vi "PUT_gear_change.vi"(8 "API Key":string="0", 9 "Cluster":cluster{"gear":string}) -> (0 "headers":string="0\r\nContent-Length: 58\r\nConnection: close\r\n\r\n", 1 "JSON string":string="0", 2 "gear":cluster{"gear":string})   [LabVIEW 2024]
uses:
  <vilib>/httpClient/PUTBuffer.vi
  <vilib>/httpClient/LabVIEWHTTPClient.lvlib
panel:
  out "error out json":errorcluster
  out "body":string="0"
  out "error out put":errorcluster
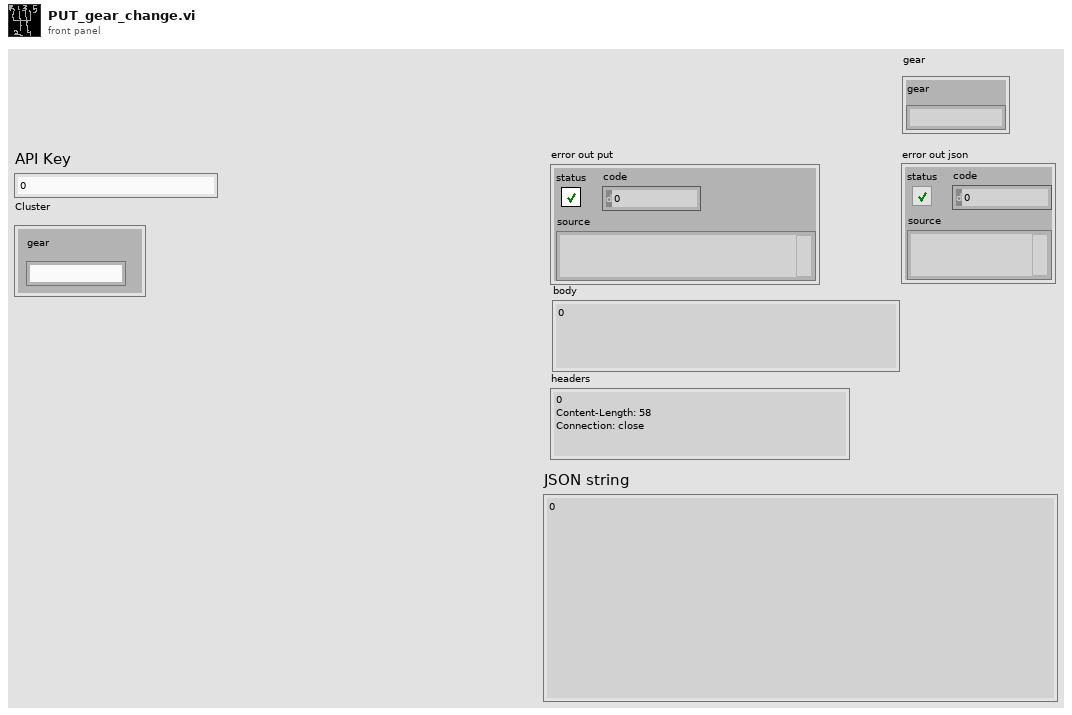
[diagram p1: front panel]
types:
  T1 = typedef "LabVIEWHTTPClient.lvlib/ClientHandle.ctl" = refnum<k1>
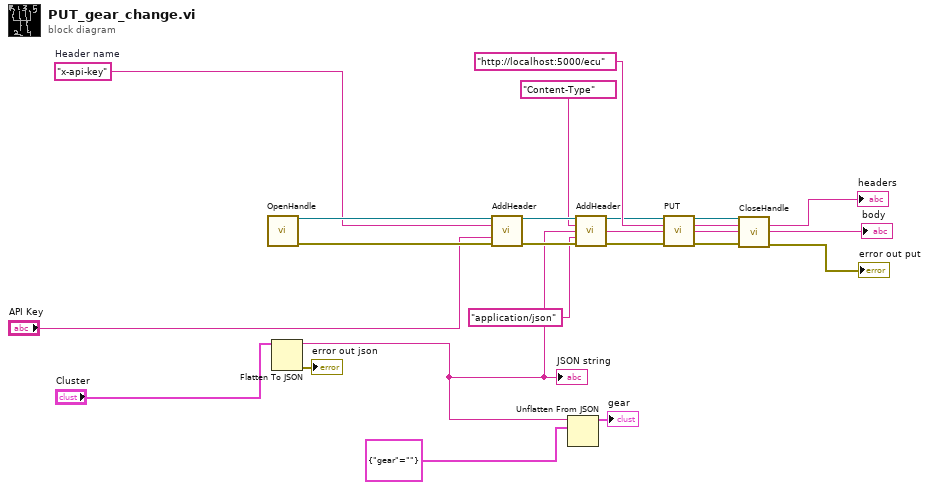
[diagram p0: block diagram]
diagram:
  w14 = "x-api-key"  # Header name
  n1 = call <vilib>:"OpenHandle.vi"() -> ("client handle out"=w15:T1, "error out"=w16:errorcluster)  [unwired: 14 in]
  n2 = Flatten To JSON(anything="Cluster") -> (JSON string=w3:string, 11:→"error out json":errorcluster)  [unwired: 2 in]
  "JSON string" <- w3
  n3 = call <vilib>:"AddHeader.vi"("client handle"=w15, "header"=w14, "value"="API Key", "error in (no error)"=w16) -> ("client handle out"=w10:T1, "error out"=w7:errorcluster)  [unwired: 10 in]
  n4 = Unflatten From JSON(JSON string=w3, type and defaults=cluster{"gear":string} {"gear"=""}) -> (value=→"gear":cluster{"gear":string})  [unwired: 5 in, 1 out]
  n5 = call <vilib>:"AddHeader.vi"("client handle"=w10, "header"="Content-Type", "value"="application/json", "error in (no error)"=w7) -> ("client handle out"=w9:T1, "error out"=w8:errorcluster)  [unwired: 10 in]
  n6 = call-poly <vilib>:"PUT.vi"("client handle"=w9, "url"="http://localhost:5000/ecu", "buffer"=w3, "error in (no error)"=w8) -> ("client handle out"=w18:T1, "headers"=→"headers":string, "body"=→"body":string, "error out"=w17:errorcluster)  [unwired: 8 in]
  n7 = call <vilib>:"CloseHandle.vi"("client handle"=w18, "error in (no error)"=w17) -> ("error out"=→"error out put":errorcluster)  [unwired: 13 in]
